vi "Is Event Refnum.vi"(10 "Self Event":refnum<data-value>) -> (2 "Error":errorcluster)   [LabVIEW 2021, in "jettl.lvlib" / "Base Queue.lvlib" / "Base Queue.lvclass"]
uses:
  Base Queue.lvclass
  Msg Strategy/Msg Strategy.lvclass
  Base Queue.lvclass/Base Queue.ctl
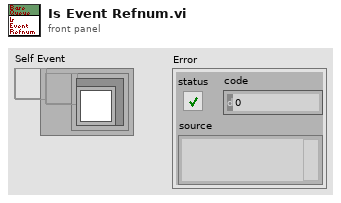
[diagram p1: front panel]
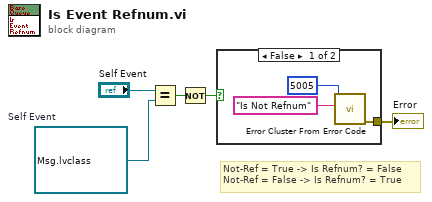
[diagram p0: block diagram]
diagram:
  w1 = refnum<data-value> refnum  # Self Event
  # "Not-Ref = True -> Is Refnum? = False\nNot-Ref = False -> Is Refnum? = True"
  n1 = Equal?(x="Self Event", y=w1) -> (x = y?=w5:bool)
  n2 = Not(x=w5) -> (.not. x?=w4:bool)
  n3 = case shown="False" w4 {
    tunnel: [w8 _] -> w3
    frame False {
      n4 = call <vilib>:"Error Cluster From Error Code.vi"("error message (\"\")"="Is Not Refnum" ("error message (\"\")"), "error code (0)"=5005) -> ("error out"=w8:errorcluster)  [unwired: 7 in]
    }
    frame True {
    }
  }
  "Error" <- w3
